vi "Set Camera Configuration.vi"(8 "error in (no error)":errorcluster, 11 "CCDCamera in":refnum<class "Simulated_CCD_Camera.lvclass">) -> (0 "error out":errorcluster, 3 "CCDCamera out":refnum<class "Simulated_CCD_Camera.lvclass">)   [LabVIEW 2018, in "Simulated_CCD_Camera.lvclass"]
uses:
  Simulated_CCD_Camera.lvclass
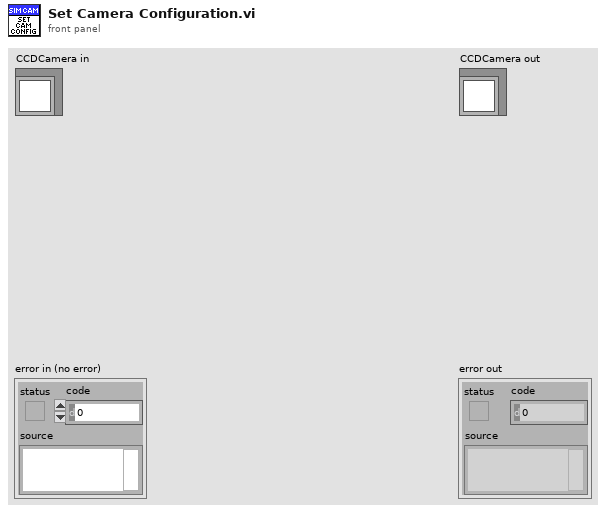
[diagram p1: front panel]
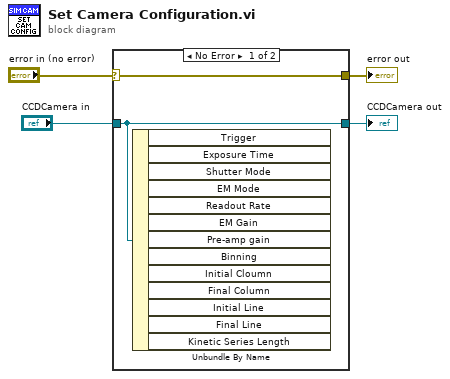
[diagram p0: block diagram]
diagram:
  n1 = case shown="No Error" "error in (no error)" {
    selector: "error in (no error)" -> [w5 w8]
    tunnel: [w5 w8] -> w4
    tunnel: [w6 w7] -> w3
    tunnel: "CCDCamera in" -> [w6 w7]
    frame No Error {
      n2 = Unbundle By Name(w6) -> ()  [unwired: 13 out]
    }
    frame Error {
    }
  }
  "error out" <- w4
  "CCDCamera out" <- w3
